vi "WSVCAP SHL Host LL RFFE Convert Channel Bytes to Bit Array.vi"(0 "RFFE Data [DUT Ordered]":u8[][](array[numeric]) format="%02x", 7 "Cycle CMD Lengths Out (bits)":u8[](array[numeric]), 9 "Cycle CMD Delay Out (ticks)":u32[](array[numeric])) -> (4 "Write Data":u64[](array[numeric]) format="%08x")   [LabVIEW 2012]
panel:
  # "0"
  # "7"
  # "0"
  # "1"
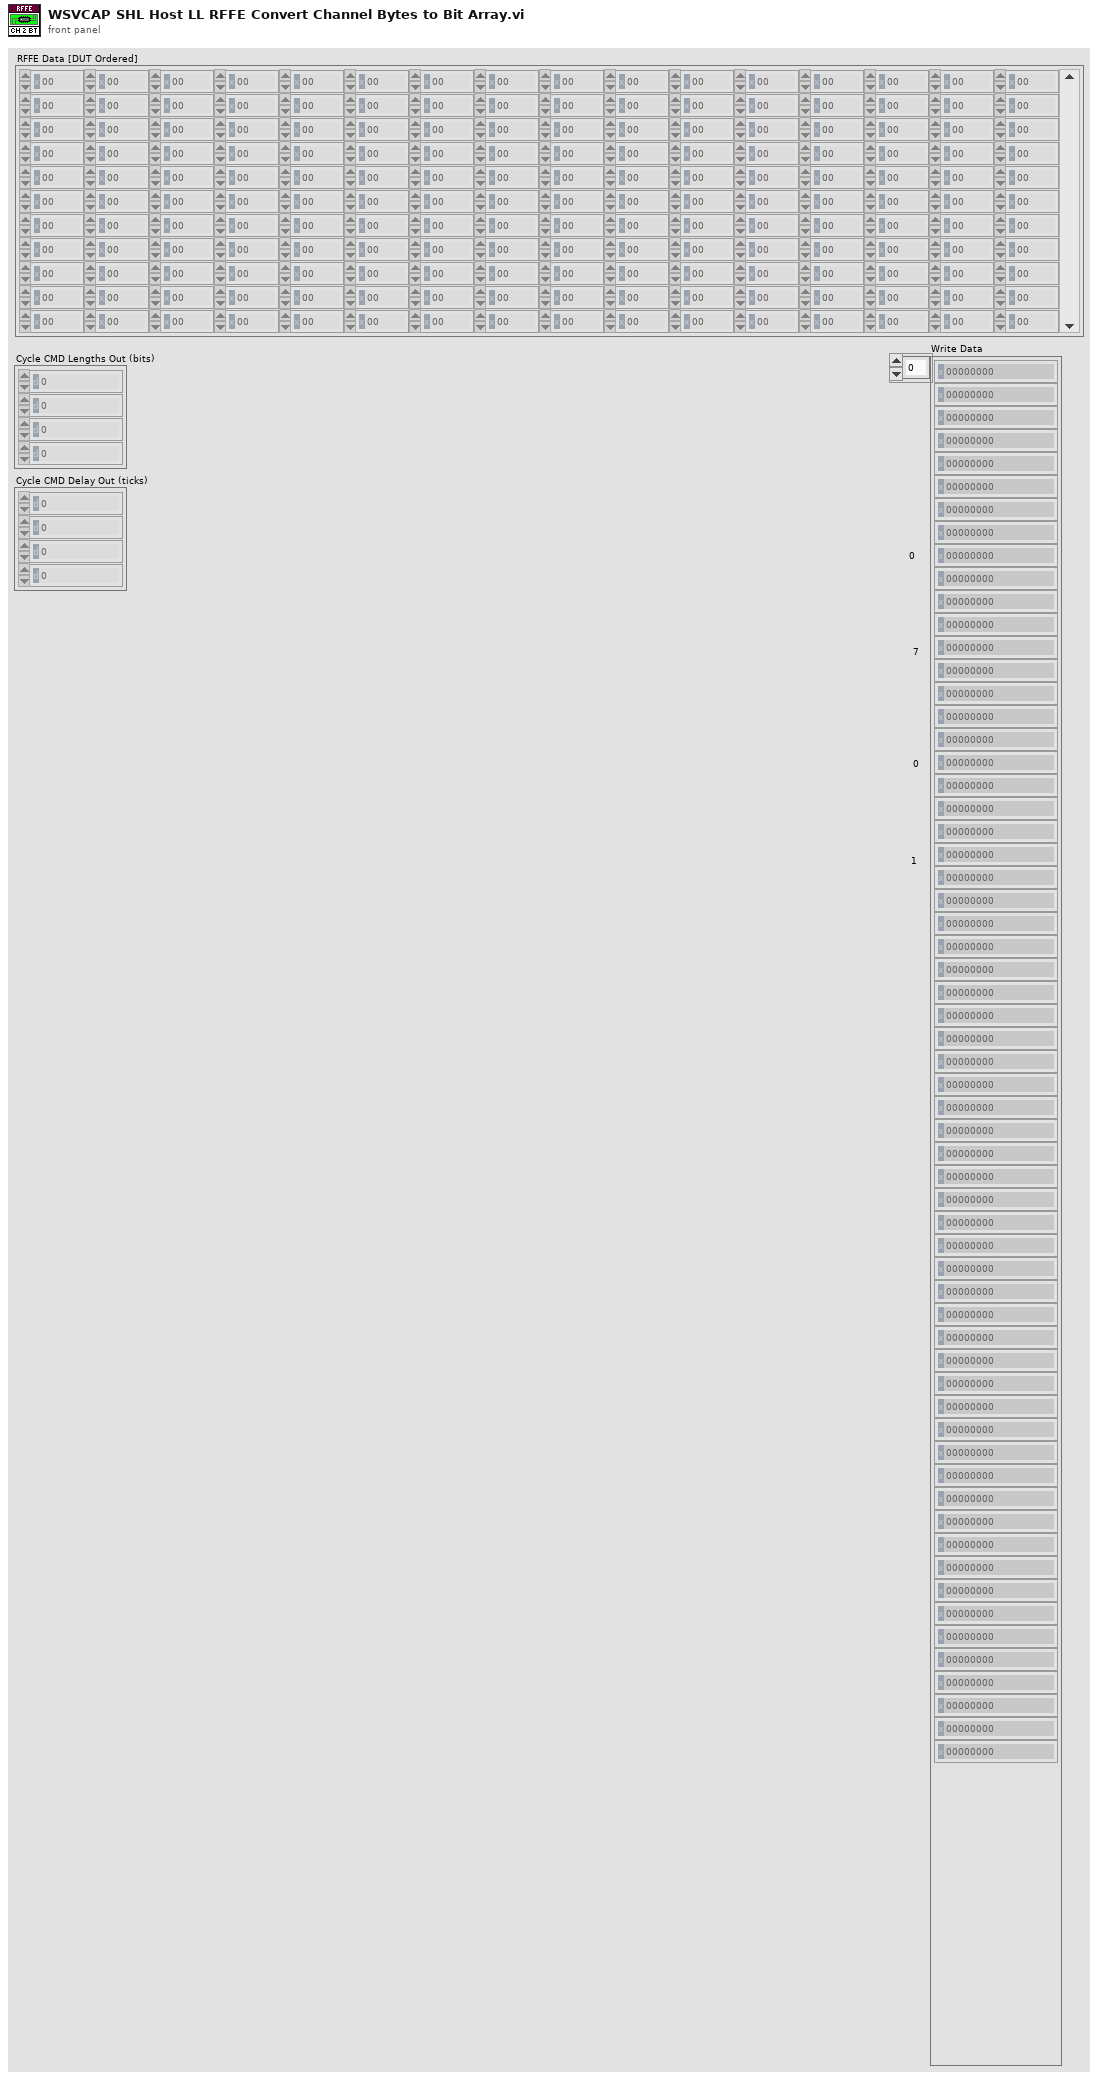
[diagram p1: front panel]
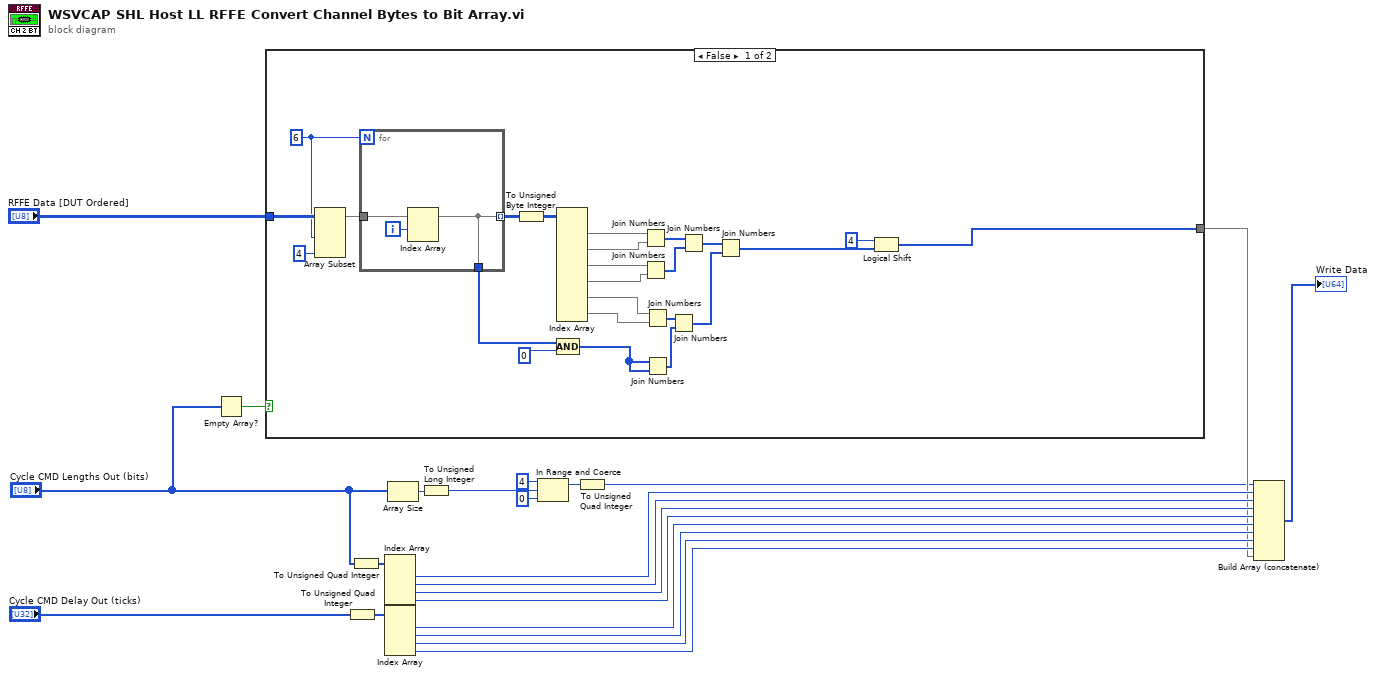
[diagram p0: block diagram]
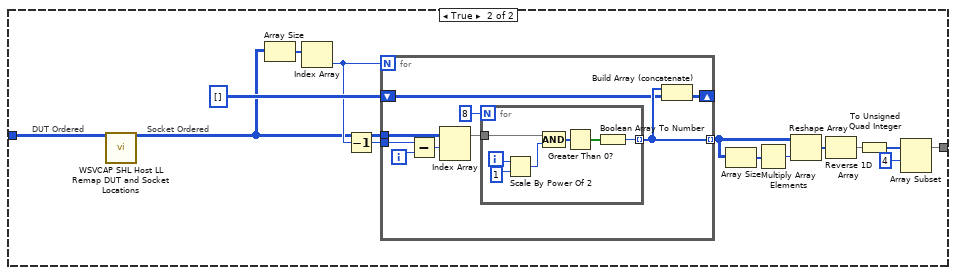
[diagram p2: hidden frame]
diagram:
  n1 = Empty Array?(array="Cycle CMD Lengths Out (bits)") -> (empty?=w3:bool)
  n2 = case shown="False" w3 {
    tunnel: "RFFE Data [DUT Ordered]" -> [w33 w54]
    tunnel: [w24 w51] -> w5
    frame False {
      w31 = 6
      n3 = Array Subset(array=w33, length (row)=w31, length (col)=4 ("length")) -> (w32:u8[][])  [unwired: 2 in]
      n4 = for {
        N: w31 -> [_]
        tunnel: w32 -> [w49]
        tunnel: [w47] -> w34 mode=indexing
        tunnel: [w47] -> w29
        i -> [w48]
        n5 = Index Array(array=w49, index (row)=w48) -> (element=w47:u8[])  [unwired: 1 in]
      }
      n6 = To Unsigned Byte Integer(number=w34) -> (unsigned 8bit integer=w39:u8[][])
      n7 = Index Array(array=w39) -> (element #1=w46:u8[], element #2=w45:u8[], element #3=w44:u8[], element #4=w43:u8[], element #5=w38:u8[], element #6=w26:u8[])  [unwired: 12 in]
      n8 = Compound Arithmetic op=AND(w29, u8 0 ("Read Data")) -> (w28:u8[])
      n9 = Join Numbers(hi=w46, lo=w45) -> ((hi.lo)=w42:u16[])
      n10 = Join Numbers(hi=w44, lo=w43) -> ((hi.lo)=w41:u16[])
      n11 = Join Numbers(hi=w38, lo=w26) -> ((hi.lo)=w37:u16[])
      n12 = Join Numbers(hi=w28, lo=w28) -> ((hi.lo)=w36:u16[])
      n13 = Join Numbers(hi=w37, lo=w36) -> ((hi.lo)=w35:u32[])
      n14 = Join Numbers(hi=w42, lo=w41) -> ((hi.lo)=w40:u32[])
      n15 = Join Numbers(hi=w40, lo=w35) -> ((hi.lo)=w25:u64[])
      n16 = Logical Shift(y=i16 4, x=w25) -> (x << y=w24:u64[])
    }
    frame True {
      # "Socket Ordered"
      # "DUT Ordered"
      n17 = call "WSVCAP SHL Host LL Remap DUT and Socket Locations.vi"("C1 DUT Ordered Data In"=w54) -> ("C1 Socket Ordered Data Out"=w53:u8[][])  [unwired: 13 in, 5 out]
      n18 = Array Size(array=w53) -> (size(s)=w59:i32[])
      n19 = Index Array(array=w59) -> (element=w57:i32)  [unwired: 1 in]
      n20 = Decrement(x=w57) -> (x-1=w56:i32)
      n21 = for {
        N: w57 -> [_]
        tunnel: w53 -> [w68]
        tunnel: [w71] -> w63 mode=indexing
        shift-right: [w70] -> _
        shift-left: u32[][] [] -> [w69]
        tunnel: w56 -> [w64]
        i -> [w66]
        n22 = Subtract(x=w64, y=w66) -> (x-y=w65:i32)
        n23 = Index Array(array=w68, index (row)=w65) -> (element=w67:u8[])  [unwired: 1 in]
        n24 = for {
          N: 8 -> [_]
          tunnel: w67 -> [w75]
          tunnel: [w74] -> w71 mode=indexing
          i -> [w77]
          n25 = Scale By Power Of 2(n=w77, x=u8 1) -> (x*2^n=w78:u8)
          n26 = Compound Arithmetic op=AND(w75, w78) -> (w79:u8[])
          n27 = Greater Than 0?(x=w79) -> (x > 0?=w73:bool[])
          n28 = Boolean Array To Number(Boolean array=w73) -> (number=w74:u32)
        }
        n29 = Build Array (concatenate)(w71, w69) -> (w70:u32[][])
      }
      n30 = Array Size(array=w63) -> (size(s)=w62:i32[])
      n31 = Multiply Array Elements(1:w62) -> (0:w61:i32)
      n32 = Reshape Array(w63, w61) -> (w58:u32[])
      n33 = Reverse 1D Array(array=w58) -> (reversed array=w55:u32[])
      n34 = To Unsigned Quad Integer(1:w55) -> (0:w52:u64[])
      n35 = Array Subset(array=w52, index=4) -> (w51:u64[])  [unwired: 1 in]
    }
  }
  n36 = To Unsigned Quad Integer(1:"Cycle CMD Delay Out (ticks)") -> (0:w2:u64[])
  n37 = To Unsigned Quad Integer(1:"Cycle CMD Lengths Out (bits)") -> (0:w14:u64[])
  n38 = Index Array(array=w14) -> (element #1=w16:u64, element #2=w15:u64, element #3=w13:u64, element #4=w12:u64)  [unwired: 4 in]
  n39 = Index Array(array=w2) -> (element #1=w11:u64, element #2=w10:u64, element #3=w9:u64, element #4=w8:u64)  [unwired: 4 in]
  n40 = Array Size(array="Cycle CMD Lengths Out (bits)") -> (size(s)=w21:i32)
  n41 = To Unsigned Long Integer(number=w21) -> (unsigned 32bit integer=w6:u32)
  n42 = In Range and Coerce(upper limit=u32 4, x=w6, lower limit=u32 0) -> (coerced(x)=w18:u32)  [unwired: 1 out]
  n43 = To Unsigned Quad Integer(1:w18) -> (0:w1:u64)
  n44 = Build Array (concatenate)(w1, w16, w15, w13, w12, w11, w10, w9, w8, w5) -> (→"Write Data":u64[])
